vi "VrefEnTabla.vi"(10 "Vref":dbl format="%#_13g", 11 "rangosDB in":string[][](array[string])=[["50", "140"], ["40", "130"]]) -> (3 "Vref_tabla":string[](array[string]))   [LabVIEW 2019, in "Prueba07.lvclass"]
uses:
  Prueba07.lvclass
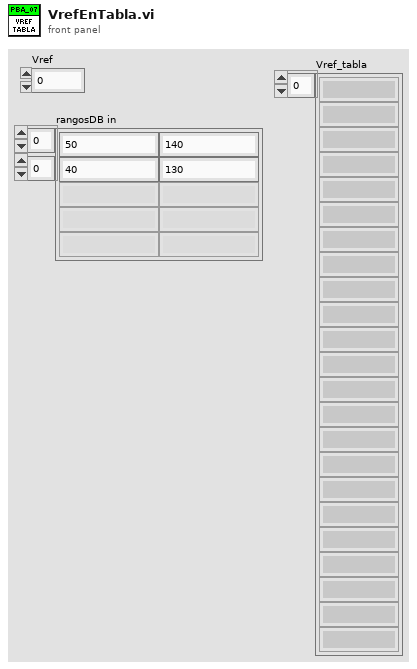
[diagram p1: front panel]
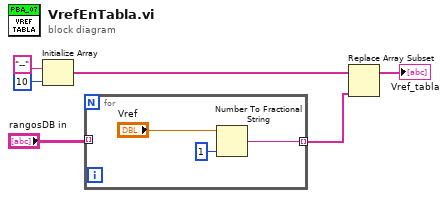
[diagram p0: block diagram]
diagram:
  n1 = Initialize Array("--" ("format string"), 10 ("dimension size")) -> (w3:string[])
  n2 = for {
    tunnel: "rangosDB in" -> [_] mode=indexing
    tunnel: [w7] -> w2 mode=indexing
    n3 = Number To Fractional String(number="Vref", precision (6)=i16 1) -> (F-format string=w7:string)  [unwired: 2 in]
  }
  n4 = Replace Array Subset(array=w3, new element=w2) -> (→"Vref_tabla":string[])  [unwired: 1 in]
